vi "PH_TKTDS-30xx.start Communication.vi"(0 "i ref in":refnum<vi>, 2 "Action":string, 5 "error in":errorcluster) -> (14 "i ref out":refnum<vi>, 19 "error out":errorcluster)   [LabVIEW 2014, in "PH_TKTDS-30xx.lvlib"]
doc: "This VI has to be set before any communication with the hardware: It sets the busy flag. It is the counterpart to \"check error\"."
uses:
  PH_TKTDS-30xx.lvlib
  PH_Basics/PH_StatusHandler/PH_StatusHandler.Status.ctl
  PH_Basics/PH_StatusHandler/PH_StatusHandler.lvlib
  PH_Basics/PH_Common/PH_Common.lvlib
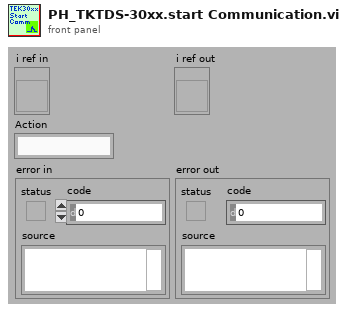
[diagram p1: front panel]
types:
  T1 = typedef "PH_TKTDS-30xx.lvlib/PH_TKTDS-30xx.i attribute.ctl" = cluster{"Default VISA Resource":string, "VISA Resource Name":refnum<visa-resource-name>, "Revision":cluster{"Instrument Driver":string, "Instrument Firmware":string}, "Selftest":cluster{"Result":u32, "Message":string}, "Channels":T2[], "Trigger Configuration":T3, "Acquisition Configuration":T4, "Fetched Waveforms":T5[], "GUI Refs":T6, "GUI Refs Channels":refnum<vi>[], "State":T7, "Error Message":string, "Allow Prdc Loop?":bool}
  T2 = typedef "PH_TKTDS-30xx.lvlib/PH_TKTDS-30xx.Channel Config.ctl" = cluster{"Channel Name":string, "Input Impedance":string, "Max Input Frequency":string, "Vertical Coupling":i32, "Channel Enabled":bool, "Probe Attenuation":dbl, "Vertical Range":dbl, "Vertical Offset":dbl}
  T3 = typedef "PH_TKTDS-30xx.lvlib/PH_TKTDS-30xx.Trigger Config.ctl" = cluster{"Source":string, "Slope":i32, "Level [V]":dbl}
  T4 = typedef "PH_TKTDS-30xx.lvlib/PH_TKTDS-30xx.Acquisition Config.ctl" = cluster{"Time base":dbl, "Record Length":u16, "Start Time":dbl, "Type":i32, "Continuous":bool}
  T5 = typedef "PH_TKTDS-30xx.lvlib/PH_TKTDS-30xx.fetched Waveform.ctl" = cluster{"Source":string, "Actual Points":u32, "Initial X":dbl, "X Increment":dbl, "Waveform Array":dbl[]}
  T6 = typedef "PH_TKTDS-30xx.lvlib/PH_TKTDS-30xx.GUI Refs.ctl" = cluster{"Trigger":refnum<vi>, "Acquisition":refnum<vi>, "Graph":refnum<vi>, "State":refnum<vi>, "Delete":refnum<vi>, "Channel to be positioned":refnum<vi>, "Postion":refnum<vi>, "Display Intensity":refnum<vi>, "VISA Resource":refnum<vi>}
  T7 = typedef "PH_StatusHandler.lvlib/PH_StatusHandler.Status.ctl" = i16
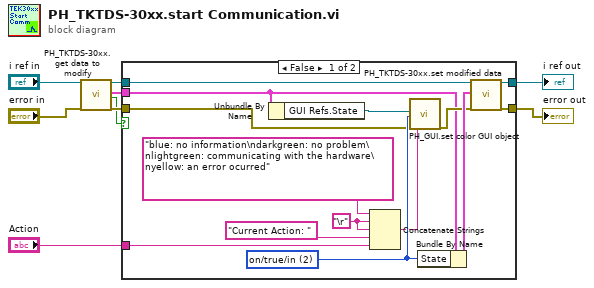
[diagram p0: block diagram]
diagram:
  n1 = call "PH_TKTDS-30xx.get data to modify.vi"("i ref in"="i ref in", "error in (no error)"="error in") -> ("i ref out"=w7:refnum<vi>, "i attribute"=w9:T1, "timed out"=w2:bool, "error out"=w8:errorcluster)  [unwired: 14 in]
  n2 = case shown="False" w2 {
    tunnel: [w23 w24] -> w6
    tunnel: w8 -> [w17 w24]
    tunnel: w7 -> [w22 w25]
    tunnel: [w21 w25] -> w4
    tunnel: w9 -> [w16 _]
    tunnel: "Action" -> [w11 _]
    frame False {
      w12 = "\r"
      w18 = T7 2 items=["no info", "off/false/out", "on/true/in", "Failure", "Alarm", "Status 1", "Status 2", "Status 3"] ("f")
      n3 = Unbundle By Name(w16) -> ("GUI Refs.State"=w15:refnum<vi>)
      n4 = Concatenate Strings("blue: no information\ndarkgreen: no problem\nlightgreen: communicating with the hardware\nyellow: an error ocurred", w12, w12, "Current Action: " ("string"), w11) -> (w13:string)
      n5 = call "PH_GUI.set color GUI object.vi"("GUI object Ref"=w15, "State"=w18, "error in (no error)"=w17, "Tip Strip (N/A)"=w13) -> ("error out"=w19:errorcluster)  [unwired: 15 in]
      n6 = Bundle By Name(cluster=w16, "State"=w18) -> (w20:T1)
      n7 = call "PH_TKTDS-30xx.set modified data.vi"("i ref in"=w22, "i attribute"=w20, "error in (no error)"=w19) -> ("i ref out"=w21:refnum<vi>, "error out"=w23:errorcluster)  [unwired: 15 in]
    }
    frame True {
    }
  }
  "error out" <- w6
  "i ref out" <- w4
